vi "Stub_ModuleName.vi"() -> (3 "Module Name":string)   [LabVIEW 2019]
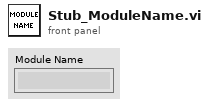
[diagram p1: front panel]
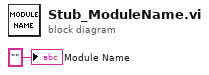
[diagram p0: block diagram]
diagram:
  "Module Name" <- ""
